vi "FilterSettings.vi"(11 "notifier":refnum<notifier>) -> ()   [LabVIEW 2013, in "main.lvlib"]
uses:
  main.lvlib
  Controls/Enum Variables.ctl
  Controls/Enum Save Action Events.ctl
panel:
  out "FilterSettingsString":string caption="String"
  in  "FilterRing":u16(ring) caption="Filter" items=["Hanning", "1 Hz Butterworth", "Moving Average 6"]
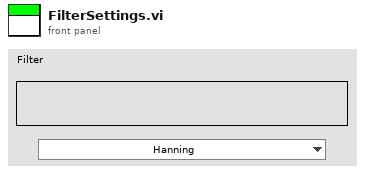
[diagram p1: front panel]
types:
  T1 = typedef "main.lvlib/Enum Variables.ctl" = enum16{"SetAcqFilter", "GetAcqFilter", "Set Filter", "Get Filter", "Set Height", "Get Height", "Set Recorded Height", "Get Recorded Height", "Set Blue Pressure", "Get Blue Pressure", "Set Red Pressure", "Get Red Pressure", "Init", "Reset Pressure", "Set Red Cursors", "Get Red Cursors", "Set Blue Cursors", "Get Blue Cursors", "Set Language", "Get Language", "Set Active Graphs", "Get ActiveGraphs", "Set Method", "Get Method", "Set Encryption", "Get Encryption", "Set ExcelVersion", "Get ExcelVersion", "Set DICOM Avail", "Get DICOM Avail", "Set DICOM Encode", "Get DICOM Encode", "Set JournalExport", "Get JournalExport", "Set Sequence", "Get Sequence", "Set DAQ Connected", "Get DAQ Connected", "Set Current Graph", "Get Current Graph", "Set General Settings", "Get Hyphenation", "Set Arm Calc Method", "Get Arm Calc Method", "Set Dicom Tags", "Get Dicom Tags", "Set BT Serial", "Get BT Serial", "Set BT Accepted Serials", "Get BT Accepted Serials", "Get BT License", "Set BT License"}
  T2 = typedef "main.lvlib/Enum Save Action Events.ctl" = enum16{"LoadReportPath", "SaveReportPath", "Load Graph Path", "Save Graph Path", "LoadDataPath", "SaveDataPath", "Load Template Path", "Save Template Path", "Load PressureFactor", "Save PressureFactor", "Init", "Load Listbox", "Save Listbox", "LoadHospInfo", "SaveHospInfo", "Load DICOM Activation", "Save DICOM Activation", "LoadDICOMInfoWL", "SaveDICOMInfoWL", "LoadDICOMInfoPACS", "SaveDICOMInfoPACS", "Load ArmCalcMethod", "Save ArmCalcMethod", "LoadItemTags", "SaveItemTags", "LoadDICOMEncoding", "SaveDICOMEncoding", "LoadJournalType", "SaveJournalType", "LoadAcqFilterType", "SaveAcqFilterType", "Load Sequence", "Save Sequence", "Load Acquisition Mode", "Save Acquisition Mode", "Load General Settings", "Save General Settings", "Load Language", "Save Language", "Load Dicom Tags", "Save Dicom Tags", "Load BT Serial", "Save BT Serial", "Load BT License", "Save BT License"}
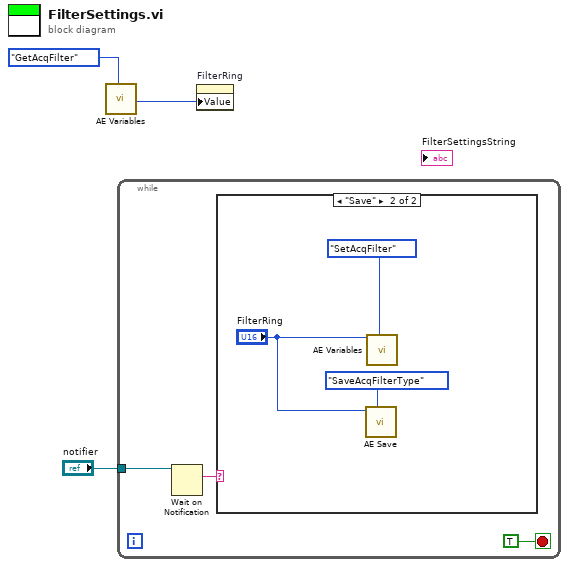
[diagram p0: block diagram]
diagram:
  n1 = call "AE Variables.vi"("Action"=Enum_Variables."GetAcqFilter") -> ("RingOut"=w1:u16)  [unwired: 11 in, 7 out]
  n2 = while {
    tunnel: "notifier" -> [w5]
    stop <- TRUE stop-if-true
    n3 = Wait on Notification(notifier=w5) -> (notification=w6:string)  [unwired: 3 in, 3 out]
    n4 = case shown="\"Save\"" w6 {
      frame "Cancel", Default {
      }
      frame "Save" {
        n5 = call "AE Save.vi"("Variant In"="FilterRing", "Action"=Enum_Save_Action_Events."SaveAcqFilterType") -> ()  [unwired: 7 in, 2 out]
        n6 = call "AE Variables.vi"("VariantIn"="FilterRing", "Action"=Enum_Variables."SetAcqFilter") -> ()  [unwired: 10 in, 8 out]
      }
    }
  }
  n7 = property on="FilterRing" class="Ring (strict)"("Value"=w1) -> ()  [unwired: 2 in, 2 out]
